vi "Test App Error Handler is Configured for Nested Process.vi"(8 "error in (no error)":errorcluster, 11 "Rig Test In":refnum<class "Application Test.lvclass">) -> (0 "error out":errorcluster, 3 "Rig Test Out":refnum<class "Application Test.lvclass">)   [LabVIEW 2020, in "Application Test.lvclass"]
uses:
  Application Test.lvclass
  C:/Program Files (x86)/National Instruments/LabVIEW 2020/vi.lib/Asteme/LUnit/Test Case.lvclass
  Mock Error Handler/Mock Error Handler.lvclass
  C:/Users/anton/Documents/GitHub/Triarc-Framework/source/Framework/Error Handler Interface/Error Handler Interface.lvclass
  Mock Process/Mock Process.lvclass
  C:/Users/anton/Documents/GitHub/Triarc-Framework/source/Framework/Process/Process.lvclass
  Framework/Application/Application.lvclass
  Framework/Process/Process.lvclass/Process.ctl
  Framework/Application/Application.lvclass/Application.ctl
  <vilib>/Asteme/LUnit/Test Case.lvclass/Test Case.ctl
  <vilib>/Asteme/LUnit/LUnit Assertion Result.lvclass/LUnit Assertion Result.ctl
  Framework/Application/Private/Add Process to Map.vi
  Framework/Application/Private/Start Idle Processes if Running.vi
  Framework/Process/Protected/Messaging/Enqueue Message.vi
  Framework/Process/Public/Lifecycle/Get Lifecycle State.vi
  Framework/Process/Protected/SubVIs/Set Context.vi
  Framework/Process/Protected/Messaging/Request Message.vi
  <vilib>/Asteme/LUnit/Palette/Pass.vi
  <vilib>/Asteme/LUnit/Palette/Fail.vi
  <vilib>/Asteme/LUnit/Variant to string.vi
  <vilib>/Asteme/LUnit/Set Assertion Type.vi
  Framework/Process/Private/SubVIs/Wait for finish.vi
  Framework/Process/Private/SubVIs/Set Lifecycle State.vi
  <vilib>/Utility/error.llb/Clear Errors.vi
  Framework/Process/Public/Lifecycle/Leave Process Loop.vi
  Framework/Process/Private/SubVIs/Enqueue Request Message.vi
  <vilib>/Asteme/LUnit/Add test result.vi
  <vilib>/Asteme/LUnit/LUnit Write Passed.vi
  <vilib>/Asteme/LUnit/LUnit Get Test Case.vi
  <vilib>/Asteme/LUnit/Assertion Result/LUnit Get Test Name.vi
  <vilib>/Asteme/LUnit/LUnit Write Message.vi
  <vilib>/Asteme/LUnit/LUnit Write Description.vi
  <vilib>/Asteme/LUnit/LUnit Write Assertion Type.vi
  <vilib>/Asteme/LUnit/Read Test Case Name.vi
  <vilib>/Utility/error.llb/Error Cluster From Error Code.vi
  Framework/Application/Private/Update Context for Owned Processes.vi
  Framework/Process/Private/SubVIs/Wait for Response Message.vi
  <vilib>/Utility/Data Type/Get Type Information.vi
  <vilib>/Utility/LVClass/Get LV Class Name.vi
  Framework/Process/Process.lvclass
  <vilib>/Asteme/LUnit/LUnit Assertion Result.lvclass
  <vilib>/Asteme/LUnit/Test Case.lvclass
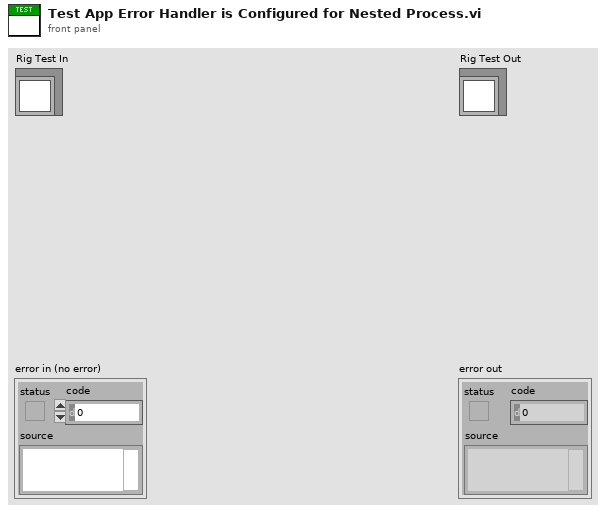
[diagram p1: front panel]
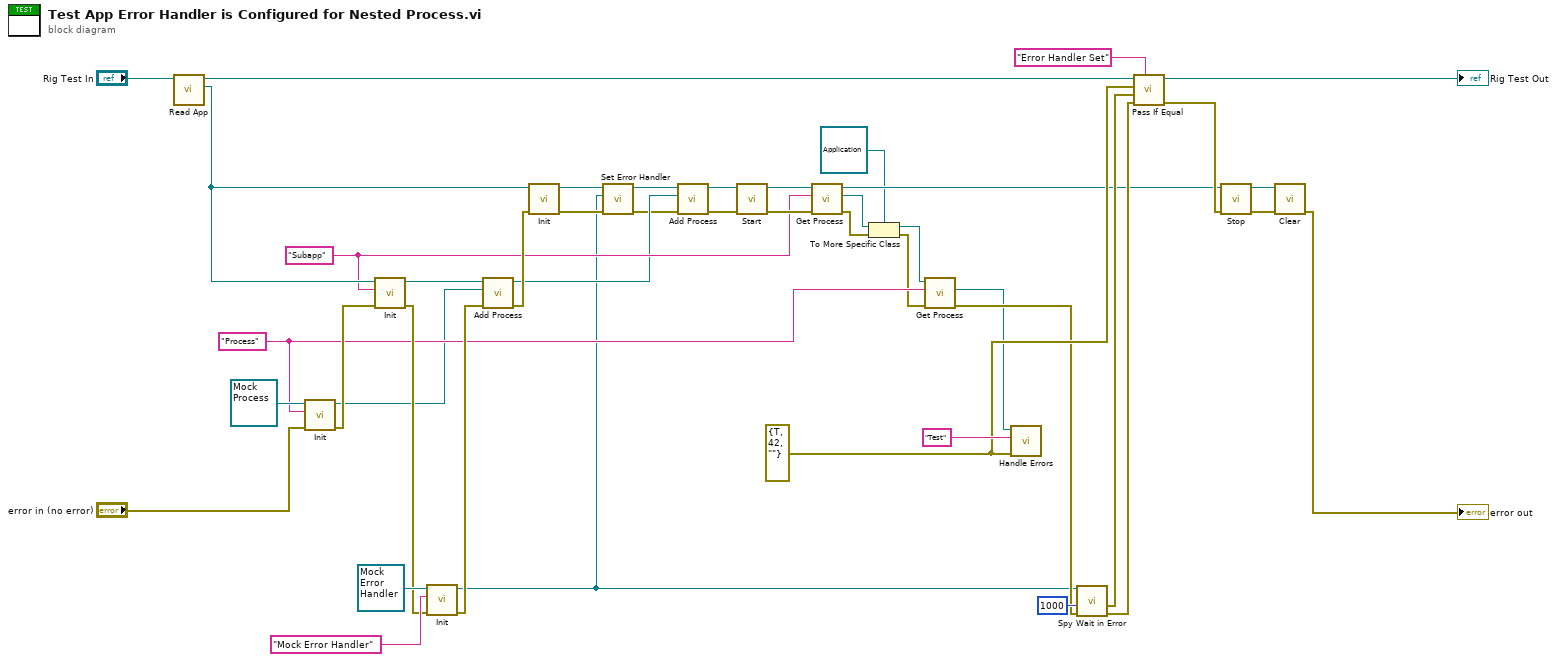
[diagram p0: block diagram]
diagram:
  w11 = "Subapp" ("Name")
  w31 = errorcluster {"status"=TRUE, "code"=42, "source"=""} ("error in (no error)")
  w26 = "Process" ("Name")
  n1 = call "Read App.vi"("Application Test In"="Rig Test In") -> ("App out"=w18:refnum<class "Application.lvclass">, "Application Test Out"=w40:refnum<class "Application Test.lvclass">)  [unwired: 8 in, 1 out]
  n2 = call-dynamic "Init.vi"("error in (no error)"="error in (no error)", "Name"=w26, "Mock Process In"=refnum<class "Mock Process.lvclass"> refnum ("Mock Process.lvclass")) -> ("error out"=w35:errorcluster, "Mock Process Out"=w24:refnum<class "Mock Process.lvclass">)  [unwired: 7 in]
  n3 = call-dynamic "Init.vi"("error in (no error)"=w35, "Name"=w11, "Process In"=w18) -> ("error out"=w34:errorcluster, "Process Out"=w43:refnum<class "Application.lvclass">)  [unwired: 7 in]
  n4 = call-dynamic "Init.vi"("error in (no error)"=w34, "Name"="Mock Error Handler", "Mock Error Handler In"=refnum<class "Mock Error Handler.lvclass"> refnum ("Mock Error Handler.lvclass")) -> ("error out"=w38:errorcluster, "Mock Error Handler Out"=w1:refnum<class "Mock Error Handler.lvclass">)  [unwired: 7 in]
  n5 = call "Add Process.vi"("error in (no error)"=w38, "Process"=w24, "Rig In"=w43) -> ("error out"=w14:errorcluster, "Rig Out"=w6:refnum<class "Application.lvclass">)  [unwired: 7 in]
  n6 = call-dynamic "Init.vi"("error in (no error)"=w14, "Process In"=w18) -> ("error out"=w13:errorcluster, "Process Out"=w3:refnum<class "Application.lvclass">)  [unwired: 8 in]
  n7 = call "Set Error Handler.vi"("error in (no error)"=w13, "Error Handler"=w1, "Process In"=w3) -> ("error out"=w4:errorcluster, "Process Out"=w2:refnum<class "Application.lvclass">)  [unwired: 7 in]
  n8 = call "Add Process.vi"("error in (no error)"=w4, "Process"=w6, "Rig In"=w2) -> ("error out"=w23:errorcluster, "Rig Out"=w20:refnum<class "Application.lvclass">)  [unwired: 7 in]
  n9 = call "Start.vi"("error in (no error)"=w23, "Process In"=w20) -> ("error out"=w21:errorcluster, "Process Out"=w19:refnum<class "Application.lvclass">)  [unwired: 8 in]
  n10 = call "Get Process.vi"("error in (no error)"=w21, "Process Name"=w11, "Rig In"=w19) -> ("error out"=w8:errorcluster, "App Process"=w9:refnum<class "Process.lvclass">, "Rig Out"=w12:refnum<class "Application.lvclass">)  [unwired: 6 in]
  n11 = To More Specific Class(target class=refnum<class "Application.lvclass"> refnum ("Rig Out"), reference=w9, error in=w8) -> (specific class reference=w5:refnum<class "Application.lvclass">, error out=w7:errorcluster)
  n12 = call "Get Process.vi"("error in (no error)"=w7, "Process Name"=w26, "Rig In"=w5) -> ("error out"=w27:errorcluster, "App Process"=w25:refnum<class "Process.lvclass">)  [unwired: 6 in, 1 out]
  n13 = call-dynamic "Handle Errors.vi"("error in (no error)"=w31, "Location"="Test", "Process In"=w25) -> ()  [unwired: 7 in, 2 out]
  n14 = call "Spy Wait in Error.vi"("error in (no error)"=w27, "timeout in ms (-1)"=1000, "Mock Error Handler In"=w1) -> ("error out"=w29:errorcluster, "Errors"=w30:errorcluster)  [unwired: 4 in, 3 out]
  n15 = call <vilib>:"Pass If Equal.vi"("Description"="Error Handler Set", "error in (no error)"=w29, "Actual"=w30, "Expected"=w31, "Test Case In"=w40) -> ("error out"=w16:errorcluster, "Test Case Out"=→"Rig Test Out":refnum<class "Application Test.lvclass">)  [unwired: 5 in]
  n16 = call "Stop.vi"("error in (no error)"=w16, "Process In"=w12) -> ("error out"=w17:errorcluster, "Process Out"=w22:refnum<class "Application.lvclass">)  [unwired: 7 in, 1 out]
  n17 = call-dynamic "Clear.vi"("error in (no error)"=w17, "Application In"=w22) -> ("error out"=→"error out":errorcluster)  [unwired: 9 in]
